vi "transition.vi"(8 "error in (no error)":errorcluster, 10 "ContextData In":refnum<class "ContextData.lvclass">, 11 "Run in":refnum<class "Win.lvclass">) -> (0 "error out":errorcluster, 2 "ContextData Out":refnum<class "ContextData.lvclass">, 3 "Next Step":refnum<class "State.lvclass">)   [LabVIEW 2019, in "Win.lvclass"]
uses:
  Win.lvclass
  State/State.lvclass
  ContextData/ContextData.lvclass
  High Scores/High Scores.lvclass
  C:/Users/fflores/Documents/GitHub Projects/Simon/Simon Game/OOP States/State/State.lvclass
  Wait Event/Wait Event.lvclass
  Win.lvclass/Win.ctl
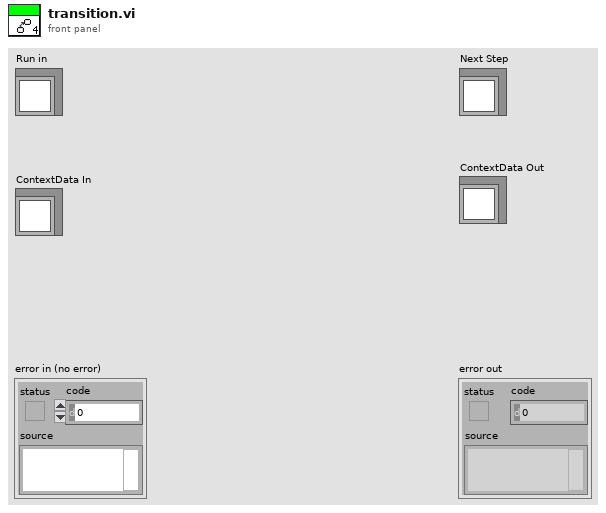
[diagram p1: front panel]
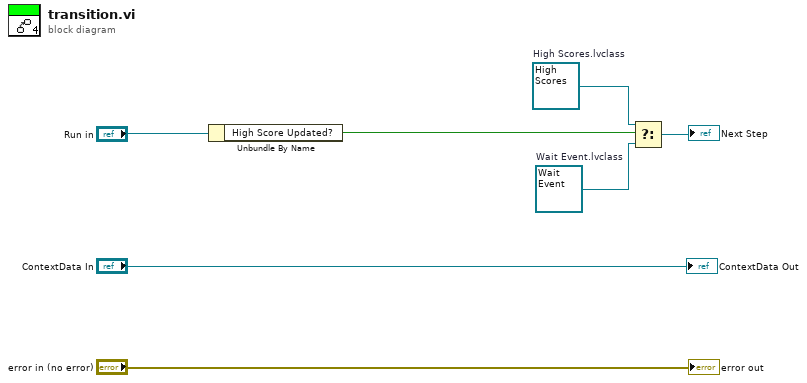
[diagram p0: block diagram]
diagram:
  w5 = refnum<class "Wait Event.lvclass"> refnum  # Wait Event.lvclass
  w6 = refnum<class "High Scores.lvclass"> refnum  # High Scores.lvclass
  n1 = Unbundle By Name("Run in") -> ("High Score Updated?"=w2:bool)
  n2 = Select(t=w6, s=w2, f=w5) -> (s? t:f=→"Next Step":refnum<class "State.lvclass">)
  "error out" <- "error in (no error)"
  "ContextData Out" <- "ContextData In"
